vi "DC_CNTRL_initialise_and_get_max_potentials.vi"(0 "Device Index":u32, 1 "Box Number":u16(ring) items=["1", "2"], 2 "Input Potentials":dbl[](array[numeric]), 3 "Current VI Path":path, 11 "error in (no error)":errorcluster) -> (4 "Handle out":u64, 12 "Current Module":i32, 14 "Max Range Array":dbl[](array[numeric]), 15 "error out":errorcluster)   [LabVIEW 2019]
uses:
  <vilib>/Utility/config.llb/Write Key (Double).vi
  <vilib>/Utility/config.llb/Read Key (Double).vi
  <vilib>/Utility/config.llb/NI_LVConfig.lvlib
panel:
  out "Device Information":T1 {"Type" items=["FT232B-FT245B", "FT8U232AM-FT8U245AM", "FT8U100AX", "UNKNOWN", "FT2232", "FT232R-FT245R", "FT2232H", "FT4232H", "FT232H"]}
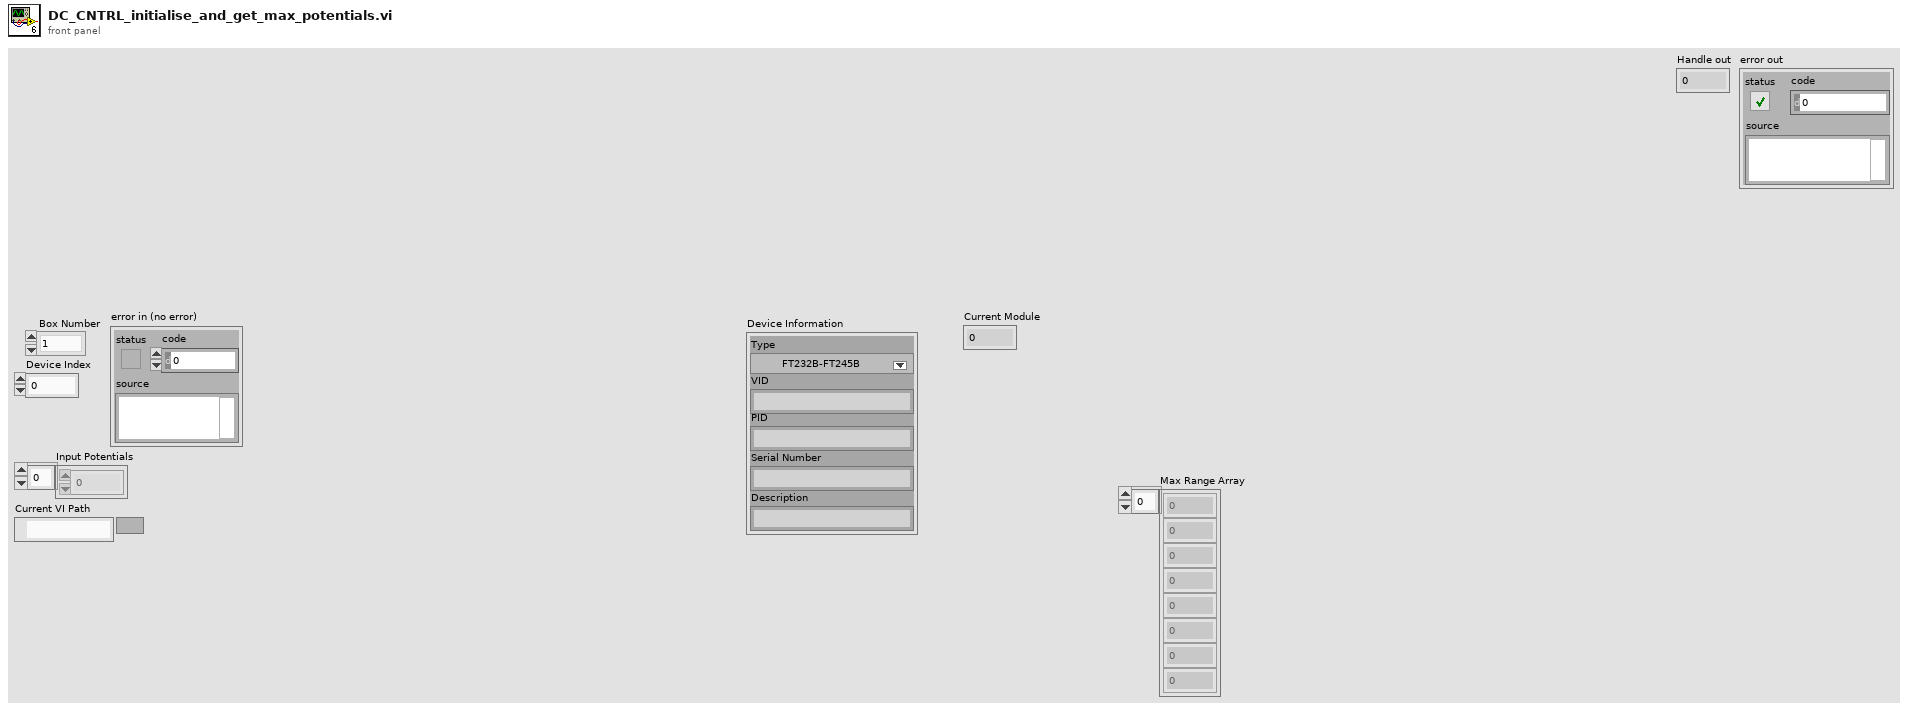
[diagram p1: front panel]
types:
  T1 = cluster{"Type":u32, "VID":string, "PID":string, "Serial Number":string, "Description":string}
  T2 = typedef "NI_LVConfig.lvlib/Config Data RefNum.ctl" = refnum<k1>
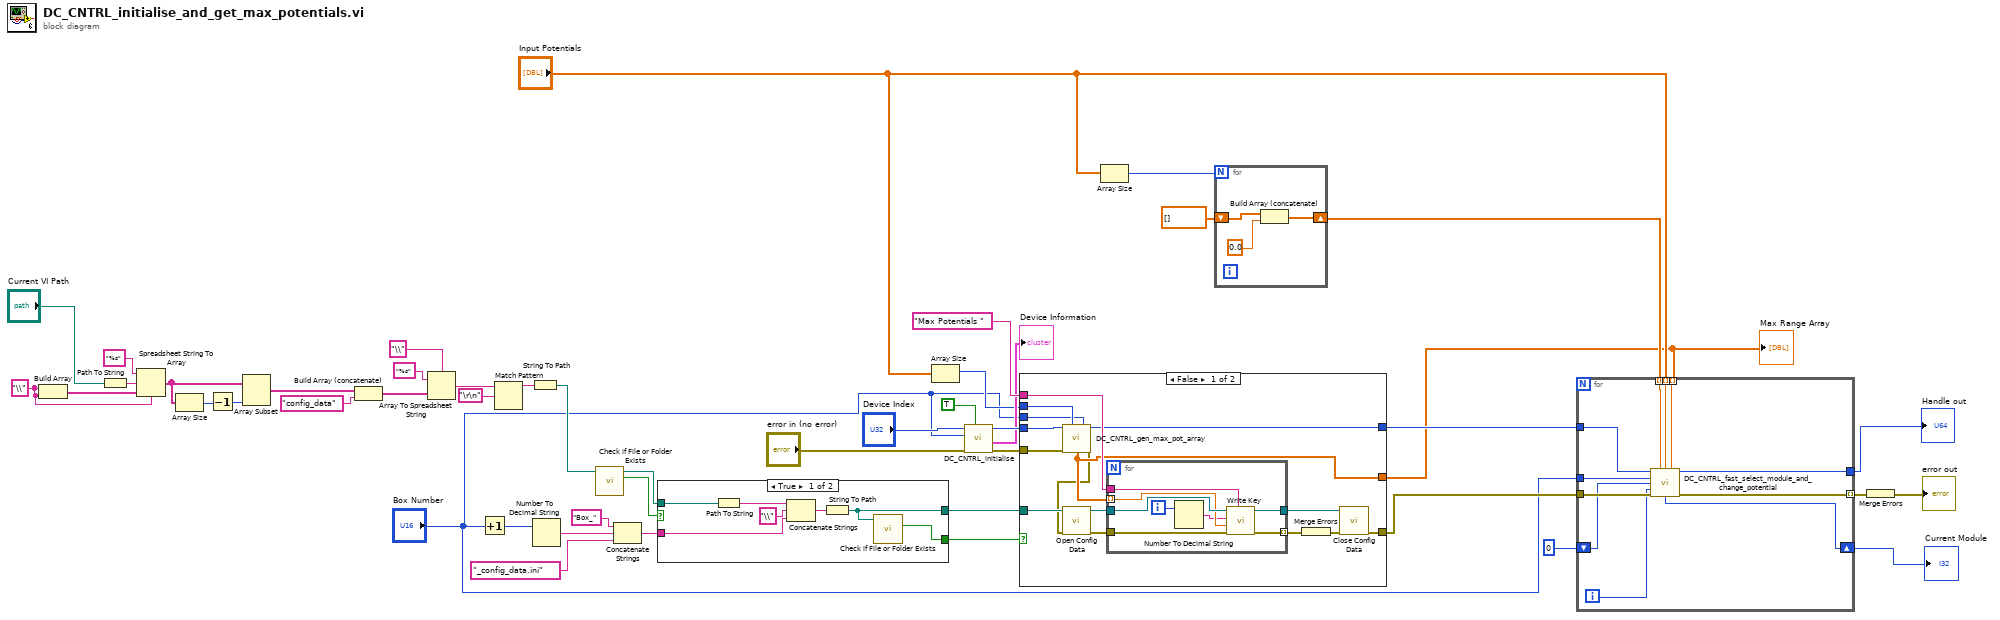
[diagram p0: block diagram]
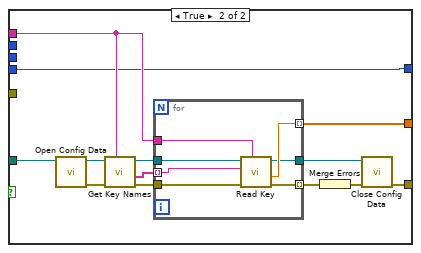
[diagram p2: hidden frame]
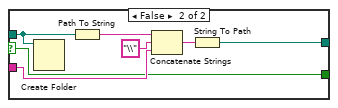
[diagram p3: hidden frame]
diagram:
  w46 = "\\" ("delimiter (Tab)")
  n1 = Build Array(w46, w46) -> (w45:string[])
  n2 = Path To String(path="Current VI Path") -> (string=w47:string)
  n3 = Spreadsheet String To Array(delimiter (Tab)=w46, format string="%s", spreadsheet string=w47, array type (2D Dbl)=w45) -> (array=w43:string[])
  n4 = Array Size(array=w43) -> (size(s)=w39:i32)
  n5 = Decrement(x=w39) -> (x-1=w42:i32)
  n6 = Array Subset(array=w43, length=w42) -> (w38:string[])  [unwired: 1 in]
  n7 = Build Array (concatenate)(w38, "config_data") -> (w36:string[])
  n8 = Array To Spreadsheet String(delimiter (Tab)="\\", array=w36, 3:"%s" ("format string")) -> (spreadsheet string=w34:string)
  n9 = Increment(x="Box Number") -> (x+1=w30:u16)
  n10 = Match Pattern(string=w34, regular expression="\r\n") -> (before substring=w33:string)  [unwired: 1 in, 3 out]
  n11 = String To Path(string=w33) -> (path=w35:path)
  n12 = Number To Decimal String(number=w30) -> (decimal integer string=w28:string)  [unwired: 1 in]
  n13 = call <vilib>:"Check if File or Folder Exists.vi"("path"=w35) -> ("file or folder exists?"=w31:bool, "dup path"=w26:path)  [unwired: 8 in, 1 out]
  n14 = Concatenate Strings("Box_", w28, "_config_data.ini") -> (w25:string)
  n15 = case shown="True" w31 {
    selector: w31 -> [_ w56]
    tunnel: w26 -> [w50 w55]
    tunnel: w25 -> [w52 w59]
    tunnel: [w49 w57] -> w23
    tunnel: [w48 w56] -> w24
    frame True {
      n16 = Path To String(path=w50) -> (string=w54:string)
      n17 = Concatenate Strings(w54, "\\" ("element"), w52) -> (w51:string)
      n18 = String To Path(string=w51) -> (path=w49:path)
      n19 = call <vilib>:"Check if File or Folder Exists.vi"("path"=w49) -> ("file or folder exists?"=w48:bool)  [unwired: 8 in, 2 out]
    }
    frame False {
      n20 = Create Folder(path (use dialog)=w55) -> ()  [unwired: 2 in, 3 out]
      n21 = Path To String(path=w55) -> (string=w61:string)
      n22 = Concatenate Strings(w61, "\\" ("element"), w59) -> (w58:string)
      n23 = String To Path(string=w58) -> (path=w57:path)
    }
  }
  n24 = Array Size(array="Input Potentials") -> (size(s)=w15:i32)
  n25 = call "DC_CNTRL_initialise.vi"("Check status?"=TRUE, "error in (no error)"="error in (no error)", "Box Number"="Box Number", "Device Index"="Device Index") -> ("error out"=w20:errorcluster, "Device Information"=→"Device Information":T1, "Handle out"=w21:u64)  [unwired: 5 in]
  n26 = case shown="False" w24 {
    tunnel: w23 -> [w76 w97]
    tunnel: [w70 w90] -> w14
    tunnel: "Max Potentials " ("section") -> [w69 w89]
    tunnel: [w68 w87] -> w8
    tunnel: w21 -> [w67 w85]
    tunnel: w20 -> [w66 _]
    tunnel: [w65 w85] -> w13
    tunnel: w15 -> [w64 _]
    tunnel: "Box Number" -> [w63 _]
    frame False {
      n27 = call "DC_CNTRL_gen_max_pot_array.vi"("Handle"=w67, "Number of supplies in box"=w64, "Box Number"=w63, "error in (no error)"=w66) -> ("Handle out"=w65:u64, "Max Range Aray"=w68:dbl[], "error out"=w62:errorcluster)  [unwired: 9 in]
      n28 = call <vilib>:"Open Config Data.vi"("error in (no error)"=w62, "configuration file path"=w76) -> ("error out"=w74:errorcluster, "refnum"=w75:T2)  [unwired: 7 in, 1 out]
      n29 = for {
        tunnel: w68 -> [w80] mode=indexing
        tunnel: w75 -> [w84]
        tunnel: w74 -> [w83]
        tunnel: [w82] -> w73
        tunnel: [w81] -> w72 mode=indexing
        tunnel: w69 -> [w77]
        i -> [w79]
        n30 = Number To Decimal String(number=w79) -> (decimal integer string=w78:string)  [unwired: 1 in]
        n31 = call-poly <vilib>:"Write Key.vi"("section"=w77, "error in (no error)"=w83, "value"=w80, "key"=w78, "refnum"=w84) -> ("error out"=w81:errorcluster, "refnum out"=w82:T2)  [unwired: 4 in, 1 out]
      }
      n32 = Merge Errors(w72) -> (w71:errorcluster)
      n33 = call <vilib>:"Close Config Data.vi"("error in (no error)"=w71, "refnum"=w73) -> ("error out"=w70:errorcluster)  [unwired: 8 in, 1 out]
    }
    frame True {
      n34 = call <vilib>:"Open Config Data.vi"("configuration file path"=w97) -> ("error out"=w95:errorcluster, "refnum"=w96:T2)  [unwired: 8 in, 1 out]
      n35 = call <vilib>:"Get Key Names.vi"("section"=w89, "error in (no error)"=w95, "refnum"=w96) -> ("error out"=w93:errorcluster, "key names"=w94:string[], "refnum out"=w86:T2)  [unwired: 5 in, 1 out]
      n36 = for {
        tunnel: w94 -> [w104] mode=indexing
        tunnel: w93 -> [w103]
        tunnel: [w102] -> w92 mode=indexing
        tunnel: [w101] -> w87 mode=indexing
        tunnel: w89 -> [w100]
        tunnel: [w99] -> w88
        tunnel: w86 -> [w98]
        n37 = call-poly <vilib>:"Read Key.vi"("section"=w100, "error in (no error)"=w103, "key"=w104, "refnum"=w98) -> ("error out"=w102:errorcluster, "value"=w101:dbl, "refnum out"=w99:T2)  [unwired: 4 in, 1 out]
      }
      n38 = Merge Errors(w92) -> (w91:errorcluster)
      n39 = call <vilib>:"Close Config Data.vi"("error in (no error)"=w91, "refnum"=w88) -> ("error out"=w90:errorcluster)  [unwired: 8 in, 1 out]
    }
  }
  "Max Range Array" <- w8
  n40 = Array Size(array="Input Potentials") -> (size(s)=w11:i32)
  n41 = for {
    N: w11 -> [_]
    shift-right: [w105] -> w9
    shift-left: dbl[] [] -> [w106]
    n42 = Build Array (concatenate)(w106, 0.0 ("element")) -> (w105:dbl[])
  }
  n43 = for {
    tunnel: w14 -> [w118]
    tunnel: w13 -> [w117]
    tunnel: "Input Potentials" -> [w116] mode=indexing
    tunnel: w9 -> [w115] mode=indexing
    tunnel: w8 -> [w114] mode=indexing
    shift-right: [w110] -> w1
    shift-left: 0 -> [w112]
    tunnel: "Box Number" -> [w111]
    tunnel: [w109] -> w5 mode=indexing
    tunnel: [w108] -> w3
    i -> [w113]
    n44 = call "DC_CNTRL_fast_select_module_and_change_potential.vi"("Handle"=w117, "Current Potential (V)"=w115, "Target Potential (V)"=w116, "Max Potential (V)"=w114, "Box Number"=w111, "Current Module Number"=w112, "Desired Module Number"=w113, "error in (no error)"=w118) -> ("Handle out"=w108:u64, "Current Module Number Out"=w110:u16, "error out"=w109:errorcluster)  [unwired: 5 in]
  }
  "Handle out" <- w3
  "Current Module" <- w1
  n45 = Merge Errors(w5) -> (→"error out":errorcluster)
